vi "SecurityAccess Sequences.vi"() -> ()   [LabVIEW 2013]
uses:
  _SubVIs/SecurityAccess_requestSeed_SubFunctions.ctl
  <vilib>/Automotive Diagnostic Command Set/Diagnostic Transport.llb/Property ID.ctl
  <vilib>/Automotive Diagnostic Command Set/Diagnostic Transport.llb/Transport Protocol Selector.ctl
  _SubVIs/SecurityAccess_requestSeed.vi
  _SubVIs/SecurityAccess_sendKey.vi
  <vilib>/Automotive Diagnostic Command Set/Diagnostic Transport.llb/Diagnostic Service.vi
  <vilib>/Automotive Diagnostic Command Set/Diagnostic Transport.llb/Apply Success Failure Error.vi
  <vilib>/addons/Automotive Diagnostic Command Set/NI_Automotive Diagnostic Command Set.lvlib
  GMLAN.lvlib
panel:
  out "error IO":errorcluster
  in  "subFunction":T1=1 items=["SPSrequestSeed"=1, "DevCtrlrequestSeed"=3]
  in  "Transmit ID":u32=2016 format="%.0x"
  in  "Receive ID":u32=2024 format="%.0x"
  in  "Baudrate":u32=500000
  in  "CAN Interface":string(combo)="CAN1"
  in  "HW select":u16(ring) items=["NI-XNET", "NI-CAN"]
  in  "UUDT Receive ID":u32=1512 format="%.0x"
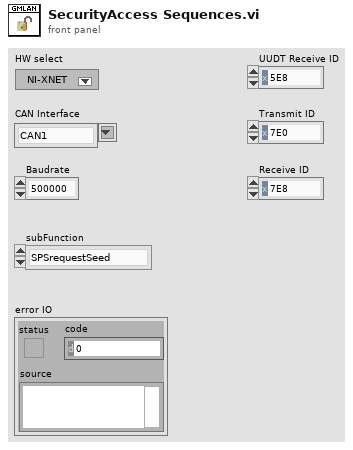
[diagram p1: front panel]
types:
  T1 = typedef "GMLAN.lvlib/SecurityAccess_requestSeed_SubFunctions.ctl" = u8
  T2 = typedef "NI_Automotive Diagnostic Command Set.lvlib/Property ID.ctl" = enum16{"Timeout Diag Command", "Timeout FC (Bs)", "Timeout CF (Cr)", "Receive Block Size (BS)", "Wait Time CF (STmin)", "Max Wait Frames (N_WFTmax)", "Wait Frames to Send (N_WAIT)", "Time between Waits (T_W)", "Fill CAN Frames", "Fill Byte", "Invalid Response as Error", "Max RspPending Count", "VWTP Command Timeout", "STmin", "P2min", "Termination"}
  T3 = typedef "NI_Automotive Diagnostic Command Set.lvlib/Transport Protocol Selector.ctl" = enum16{"ISO TP - Normal Mode", "ISO TP - Mixed Mode", "VW TP 2.0", "Diagnostics on IP", "ISO TP LIN"}
  T4 = typedef "NI_Automotive Diagnostic Command Set.lvlib/Diag Reference.ctl" = cluster{"Diag CAN Handle":u32, "Transport Protocol":T3, "Receive Address Extension":u8, "Transmit Address Extension":u8, "Receive CAN Id":u32, "Transmit CAN Id":u32, "Diag CAN Queue":refnum<queue>, "Log Frames ?":bool, "My TP Address":u8, "Other TP Address":u8, "T1":u16, "T2":u16, "T3":u16, "T4":u16, "Tx SN":u8, "Block Size":u8, "Rx SN":u8, "VW TP Initialized?":bool, "Tx block no":u8, "baud rate":u32, "Interface":string, "Channel Diag CAN Handle":u32, "UDP Connection ID":refnum<k16>, "TCP Connection ID":refnum<k5>, "Target IP Addr":u32, "Source Address":u16, "Target Address":u16, "Send Header NACK?":bool, "DLL Handle":u32, "NAD":u8, "Time Stamp read first":dbl, "Time Stamp read last":dbl, "Time Stamp write first":dbl, "Time Stamp write last":dbl}
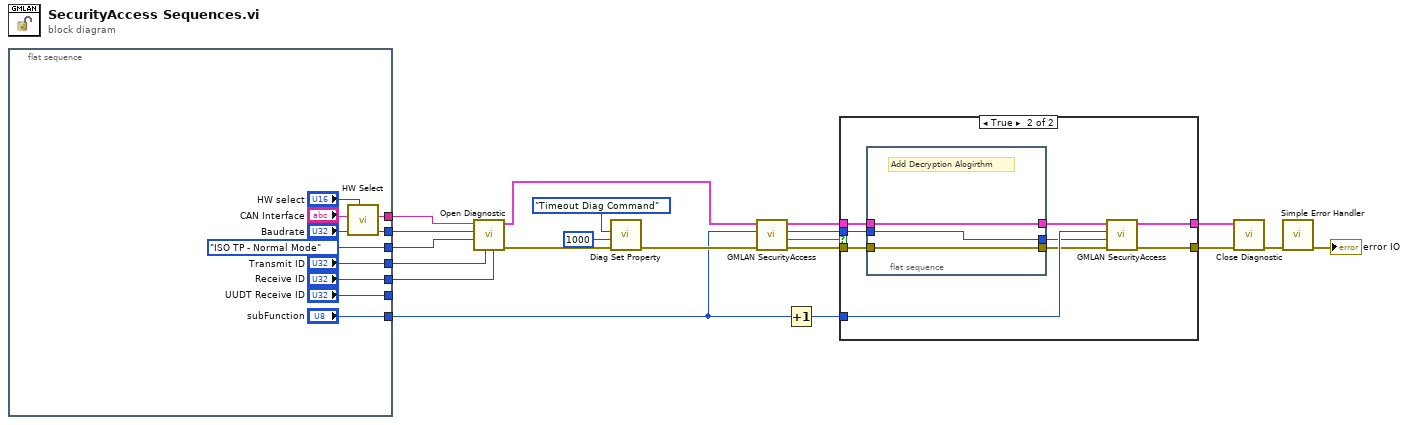
[diagram p0: block diagram]
diagram:
  n1 = flat-sequence {
    tunnel: [w29] -> w20
    tunnel: ["Baudrate"] -> w13
    tunnel: [Transport_Protocol_Selector."ISO TP - Normal Mode" ("Transport Protocol")] -> w19
    tunnel: ["Transmit ID"] -> w18
    tunnel: ["Receive ID"] -> w17
    tunnel: ["UUDT Receive ID"] -> _
    tunnel: ["subFunction"] -> w10
    frame #0 {
      n2 = call "HW Select.vi"("HW select"="HW select", "CAN port"="CAN Interface") -> ("CAN port out"=w29:string)  [unwired: 9 in]
    }
  }
  n3 = call <vilib>:"Open Diagnostic.vi"("Receive ID"=w17, "Transmit ID"=w18, "Transport Protocol"=w19, "Baud Rate"=w13, "CAN Interface"=w20) -> ("error out"=w16:errorcluster, "diag ref out"=w11:T4)  [unwired: 1 in, 4 out]
  n4 = call <vilib>:"Diag Set Property.vi"("error in (no error)"=w16, "property value"=u32 1000, "property ID"=Property_ID."Timeout Diag Command") -> ("error out"=w12:errorcluster)  [unwired: 7 in, 1 out]
  n5 = call-poly "GMLAN SecurityAccess.vi"("error in (no error)"=w12, "subFunction"=w10, "diag ref in"=w11) -> ("error out"=w8:errorcluster, "success?"=w5:bool, "SecuritySeed"=w6:u16, "diag ref out"=w7:T4)  [unwired: 5 in]
  n6 = Increment(x=w10) -> (x+1=w9:T1)
  n7 = case shown="True" w5 {
    tunnel: w9 -> [_ w40]
    tunnel: w8 -> [w31 w38]
    tunnel: w7 -> [w30 w36]
    tunnel: w6 -> [_ w35]
    tunnel: [w31 w34] -> w3
    tunnel: [w30 w33] -> w2
    frame False {
    }
    frame True {
      n8 = flat-sequence {
        tunnel: [w43] -> w39
        tunnel: w38 -> [w43]
        tunnel: [w42] -> w37
        tunnel: w36 -> [w42]
        tunnel: [w41] -> w32
        tunnel: w35 -> [w41]
        frame #0 {
          # "Add Decryption Alogirthm"
        }
      }
      n9 = call-poly "GMLAN SecurityAccess.vi"("error in (no error)"=w39, "SecuritySeed"=w32, "subFunction"=w40, "diag ref in"=w37) -> ("error out"=w34:errorcluster, "diag ref out"=w33:T4)  [unwired: 5 in, 1 out]
    }
  }
  n10 = call <vilib>:"Close Diagnostic.vi"("error in (no error)"=w3, "diag ref in"=w2) -> ("error out"=w1:errorcluster)  [unwired: 9 out]
  n11 = call <vilib>:"Simple Error Handler.vi"("error in (no error)"=w1) -> ("error out"=→"error IO":errorcluster)  [unwired: 1 in, 7 out]
